vi "1.vi"() -> ()   [LabVIEW 2019]
uses:
  <vilib>/imath/engines/lvmath/Plug In/_Char/NIMS_CH_character datatype.ctl
  <vilib>/imath/engines/lvmath2/RunTimeEngine/Managers/WorkSpace/UID Generator.vi
  <vilib>/imath/engines/lvmath2/RunTimeEngine/BuiltInFunctions/zeros/NIMS_V=zeros(I32,I32).vi
  <vilib>/imathl/engines/lvmath/Functions/Error Handling/Create Error.vi
  <vilib>/imath/engines/lvmath2/RunTimeEngine/IndexReplace/NIMS V(S)=S.vi
  <instcachedir>/0/NIMS V(S)=S_BD5C8CB81B6E4D99B8C0034EA1BEE55D.lvgen/NIMS V(S)=S_BD5C8CB81B6E4D99B8C0034EA1BEE55D_000.vi
  <vilib>/imath/engines/lvmath2/RunTimeEngine/RangeToken/NIMS_Range_R2 - Float.vi
  <instcachedir>/0/NIMS_Range_R2 - Float_E92E97654E134110B10F16A3994F6405.lvgen/NIMS_Range_R2 - Float_E92E97654E134110B10F16A3994F6405_000.vi
  <vilib>/imath/engines/lvmath2/RunTimeEngine/CommandStatement/MC_CommandStatement_break.vi
  <vilib>/imath/engines/lvmath2/RunTimeSupport/NIMS_Error if Not Equal.vi
  <instcachedir>/0/NIMS_Error if Not Equal_D50A0F08CBFC40E0B64682CCD852CBC7.lvgen/NIMS_Error if Not Equal_D50A0F08CBFC40E0B64682CCD852CBC7_000.vi
  <vilib>/imath/engines/lvmath2/RunTimeEngine/IndexRead/NIMS V(S).vi
  <instcachedir>/0/NIMS V(S)_0488751826AF41519A22953C041130DC.lvgen/NIMS V(S)_0488751826AF41519A22953C041130DC_000.vi
  <vilib>/imath/engines/lvmath2/RunTimeEngine/BuiltInFunctions/mod/NIMS_mod_no_size_check.vi
  <vilib>/imath/engines/lvmath2/RunTimeEngine/ErrorHandling/NIMS_Create Error From Enums.vi
  <vilib>/imath/engines/lvmath2/RunTimeEngine/RunTimeType/NIMS_RunTimeType_From StrictType (excl LVString).vi
  <vilib>/imath/engines/lvmath2/RunTimeEngine/LocalVariableDefStatement/MC_LocalVariableDefStatement_Display.vi
  <vilib>/imath/engines/lvmath2/RunTimeEngine/BuiltInFunctions/num_to_str/NIMS_num_to_str(GRowV,I32).vi
  <instcachedir>/0/NIMS_num_to_str(GRowV,I32)_4BA4510D64AF4E68B18295D765365DA3.lvgen/NIMS_num_to_str(GRowV,I32)_4BA4510D64AF4E68B18295D765365DA3_000.vi
  <vilib>/imath/engines/lvmath/Plug In/_Char/NIMS_CH_String to Character Array.vi
  <vilib>/imath/engines/lvmath2/RunTimeEngine/BuiltInFunctions/max/1 input/NIMS_max(RV).vi
  <instcachedir>/0/NIMS_max(RV)_237633DB1D604D5BA7001287DF3C7957.lvgen/NIMS_max(RV)_237633DB1D604D5BA7001287DF3C7957_000.vi
  <vilib>/imath/engines/lvmath2/RunTimeEngine/ErrorHandling/NIMS_Error From Error Code.vi
  <vilib>/imath/engines/lvmath2/RunTimeEngine/BuiltInFunctions/min/1 input/NIMS_min(RV).vi
  <instcachedir>/0/NIMS_min(RV)_EE2DD3E2888846108C5160A664B67832.lvgen/NIMS_min(RV)_EE2DD3E2888846108C5160A664B67832_000.vi
  <vilib>/imath/engines/lvmath2/RunTimeEngine/BuiltInFunctions/histogram/NIMS_[V]=histogram(V).vi
  <instcachedir>/0/NIMS_RunTimeType_From StrictType (excl LVString)_D8AFBA86A94845AAA577C895450664BD.lvgen/NIMS_RunTimeType_From StrictType (excl LVString)_D8AFBA86A94845AAA577C895450664BD_000.vi
  <vilib>/imath/engines/lvmath2/RunTimeEngine/BuiltInFunctions/density_kernel/NIMS_density_kernel(V,Var).vi
  <vilib>/imath/engines/lvmath2/RunTimeEngine/BuiltInFunctions/figure/NIMS_figure.vi
  <vilib>/imath/engines/lvmath2/RunTimeEngine/BuiltInFunctions/subplot/NIMS_subplot(I32, I32, I32).vi
  <vilib>/imath/engines/lvmath2/RunTimeEngine/BuiltInFunctions/plot/NIMS_plot(RM, RM, Str).vi
  <vilib>/imath/engines/lvmath/Plug In/_Char/NIMS_CH_Character RV to String.vi
  <vilib>/imath/engines/lvmath2/RunTimeEngine/BuiltInFunctions/title/NIMS_title.vi
  <vilib>/imath/engines/lvmath2/RunTimeEngine/BuiltInFunctions/hold/NIMS_hold(Enums).vi
  <vilib>/imath/engines/lvmath2/RunTimeEngine/RangeToken/NIMS_Range.vi
  <instcachedir>/0/NIMS_Range_FADF6ADDA3E145BB934C8BD4C7DAAB97.lvgen/NIMS_Range_FADF6ADDA3E145BB934C8BD4C7DAAB97_000.vi
  <vilib>/imath/engines/lvmath2/RunTimeEngine/BuiltInFunctions/size/NIMS_I32Row=size(GRow).vi
  <instcachedir>/0/NIMS_I32Row=size(GRow)_E5C05C6B13124B29B774CC4F993D3C59.lvgen/NIMS_I32Row=size(GRow)_E5C05C6B13124B29B774CC4F993D3C59_000.vi
  <vilib>/imath/engines/lvmath2/RunTimeEngine/BuiltInFunctions/ones/NIMS_M=ones(I32V).vi
  <vilib>/imath/engines/lvmath2/RunTimeEngine/BuiltInFunctions/axis/NIMS_axis.vi
  <vilib>/imath/engines/lvmath2/RunTimeEngine/Managers/SymbolTable/Clear UID.vi
  <vilib>/imath/engines/lvmath2/RunTimeEngine/NodeEndStatement/NIMS_NodeEndStatement_Output.vi
  <instcachedir>/0/NIMS_NodeEndStatement_Output_53EC0D466D134D7ABD903AC30B43404B.lvgen/NIMS_NodeEndStatement_Output_53EC0D466D134D7ABD903AC30B43404B_005.vi
  <instcachedir>/0/NIMS_NodeEndStatement_Output_53EC0D466D134D7ABD903AC30B43404B.lvgen/NIMS_NodeEndStatement_Output_53EC0D466D134D7ABD903AC30B43404B_004.vi
  <vilib>/imath/engines/lvmath2/RunTimeEngine/ErrorHandling/NIMS_Finalize Error.vi
  <vilib>/imath/engines/lvmath2/RunTimeEngine/Managers/SymbolTable/NIMS_WorkSpace.lvlib
panel:
  out "最小值":dbl
  out "最大值":dbl
  out "直方图":i32[](graph)
  out "1~4阶矩":dbl[](array[numeric])
  out "散点图":dbl[](graph)
  in  "num":dbl=1000.0
  in  "s1":dbl=12357.0
  in  "r":dbl=2045.0
  out "折线图":dbl[](graph)
  in  "b":dbl=1.0
  in  "M":dbl=1048576.0 format="%#_7f"
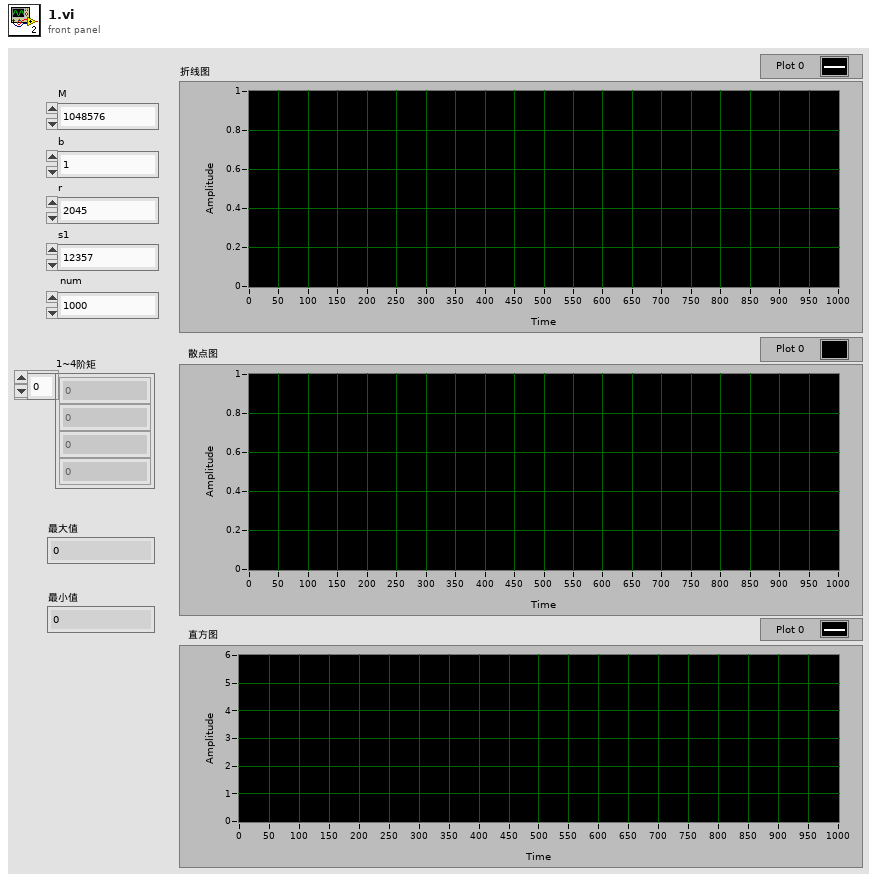
[diagram p1: front panel]
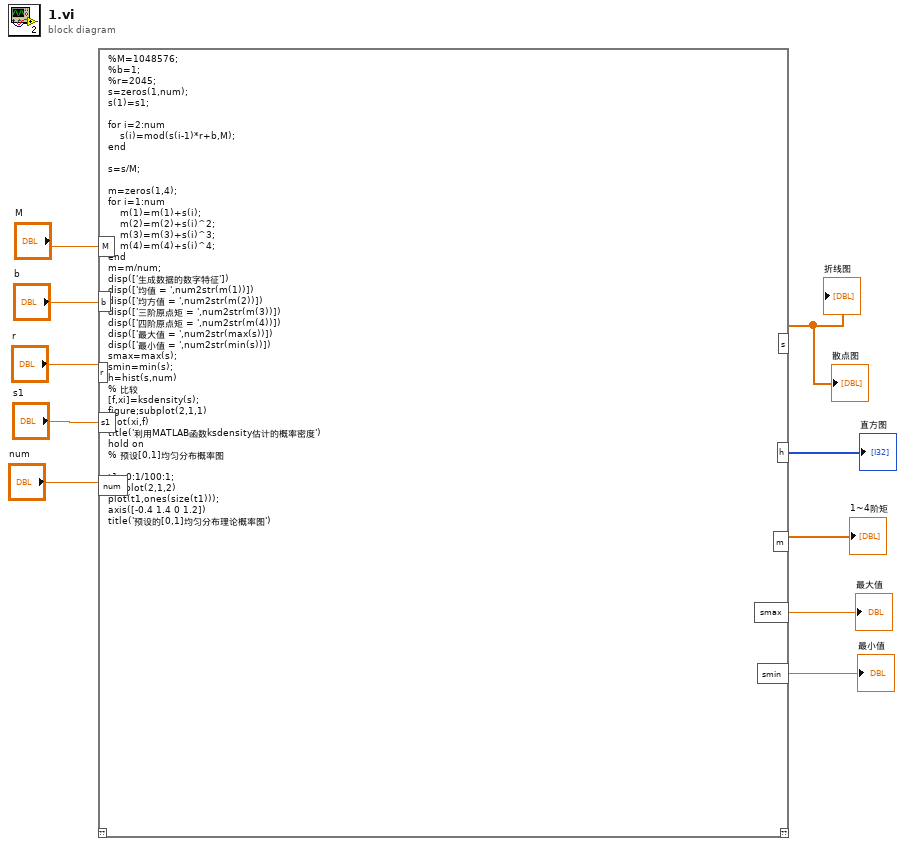
[diagram p0: block diagram]
diagram:
  n1 = mathscript code="%M=1048576;\n%b=1;\n%r=2045;\ns=zeros(1,num);\ns(1)=s1;\n\nfor i=2:num\n    s(i)=mod(s(i-1)*r+b,M);\nend\n\ns=s/M;\n\nm=zeros(1,4);\nfor i=1:num\n    m(1)=m(1)+s(i);\n    m(2)=m(2)+s(i)^2;\n    m(3)=m(3)+s(i)^3;\n    m(4)=m(4)+s(i)^4;\nend\nm=m/num;\ndisp(['生成数据的数字特征'])\ndisp(['均值 = ',num2str(m(1))])\ndisp(['均方值 = ',num2str(m(2))])\ndisp(['三阶原点矩 = ',num2str(m(3))])\ndisp(['四阶原点矩 = ',num2str(m(4))])\ndisp(['最大值 = ',num2str(max(s))])\ndisp(['最小值 = ',num2str(min(s))])\nsmax=max(s);\nsmin=min(s);\nh=hist(s,num)\n% 比较\n[f,xi]=ksdensity(s);\nfigure;subplot(2,1,1)\nplot(xi,f)\ntitle('利用MATLAB函数ksdensity估计的概率密度')\nhold on\n% 预设[0,1]均匀分布概率图\n\nt1=0:1/100:1;\nsubplot(2,1,2)\nplot(t1,ones(size(t1)));\naxis([-0.4 1.4 0 1.2])\ntitle('预设的[0,1]均匀分布理论概率图')"("M"="M", "s1"="s1", "b"="b", "r"="r", "num"="num") -> ("s"=→"折线图" →"散点图":dbl[], "h"=→"直方图":i32[], "m"=→"1~4阶矩":dbl[], "smax"=→"最大值":dbl, "smin"=→"最小值":dbl)  [unwired: 1 in, 1 out]
